vi "Untitled 4.vi"() -> ()   [LabVIEW 2015]
panel:
  out "x-y*floor(x/y)":dbl
  out "floor(x/y)":dbl
  in  "x":dbl
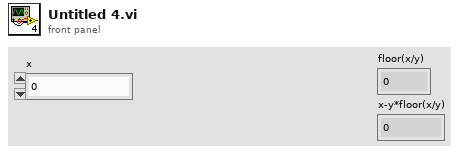
[diagram p1: front panel]
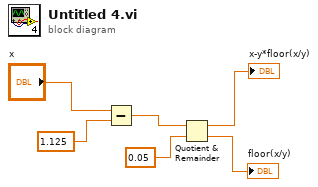
[diagram p0: block diagram]
diagram:
  n1 = Subtract(x="x", y=1.125) -> (x-y=w4:dbl)
  n2 = Quotient & Remainder(x=w4, y=0.05) -> (x-y*floor(x/y)=→"x-y*floor(x/y)":dbl, floor(x/y)=→"floor(x/y)":dbl)
